vi "Test_monitorCommand_setLogLevel.vi"(8 "error in (no error)":errorcluster, 11 "command_setLogLevel_Ctl":T1) -> (0 "error out":errorcluster, 2 "function return":i32, 3 "command_setLogLevel_Ctl out":T1)   [LabVIEW 2016, in "SALLV_Test.lvlib"]
doc: "int Test_shm_monitorCommand_setLogLevelLV(Test_command_setLogLevelLV *command_setLogLevel_Ctl );"
uses:
  SALLV_Test.lvlib
  DataTypes/command_setLogLevel.ctl
  SALLV_Test.so
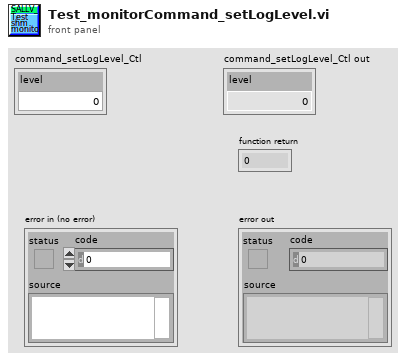
[diagram p1: front panel]
types:
  T1 = typedef "SALLV_Test.lvlib/command_setLogLevel.ctl" = cluster{"level":i32}
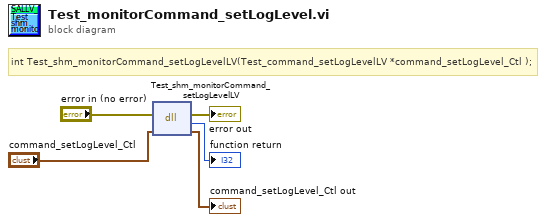
[diagram p0: block diagram]
diagram:
  # "int Test_shm_monitorCommand_setLogLevelLV(Test_command_setLogLevelLV *command_setLogLevel_Ctl );"
  n1 = dll-call lib="home/ccontaxis/Code/SALLV_Test/SALLV_Test.*" fn="Test_shm_monitorCommand_setLogLevelLV"(error in="error in (no error)", "command_setLogLevel_Ctl"="command_setLogLevel_Ctl") -> (error out=→"error out":errorcluster, →"function return":i32, "command_setLogLevel_Ctl"=→"command_setLogLevel_Ctl out":T1)  [unwired: 2 in, 1 out]
